vi "Update State.vi"(8 "error in":errorcluster, 10 "State":bool, 11 "DAQmxSwitch in":refnum<class "DAQmxSwitch.lvclass">) -> (0 "error out":errorcluster, 3 "DAQmxSwitch out":refnum<class "DAQmxSwitch.lvclass">)   [LabVIEW 2009, in "DAQmxSwitch.lvclass"]
uses:
  DAQmxSwitch.lvclass
  Switch.lvclass
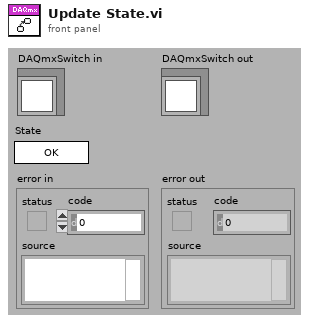
[diagram p1: front panel]
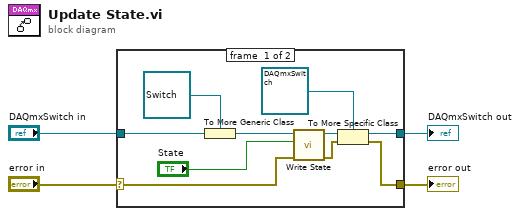
[diagram p0: block diagram]
diagram:
  n1 = case shown="No Error" "error in" {
    selector: "error in" -> [w10 w16]
    tunnel: [w6 w16] -> w3
    tunnel: [w5 w15] -> w1
    tunnel: "DAQmxSwitch in" -> [w14 w15]
    frame #0 {
      n2 = To More Generic Class(target class=refnum<class "Switch.lvclass"> refnum ("Switch.lvclass"), reference=w14) -> (generic class reference=w12:refnum<class "Switch.lvclass">)
      n3 = call-dynamic "Write State.vi"("error in (no error)"=w10, "State"="State", "Switch in"=w12) -> ("error out"=w8:errorcluster, "Switch out"=w9:refnum<class "Switch.lvclass">)  [unwired: 7 in]
      n4 = To More Specific Class(target class=refnum<class "DAQmxSwitch.lvclass"> refnum ("DAQmxSwitch in"), reference=w9, error in=w8) -> (specific class reference=w5:refnum<class "DAQmxSwitch.lvclass">, error out=w6:errorcluster)
    }
    frame #1 {
    }
  }
  "error out" <- w3
  "DAQmxSwitch out" <- w1
